vi "Subscriber.vi"() -> ()   [LabVIEW 2020]
panel:
  in  "stop":bool
  out "String":string
  out "Numeric":dbl
  out "Boolean":bool
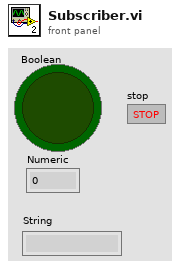
[diagram p1: front panel]
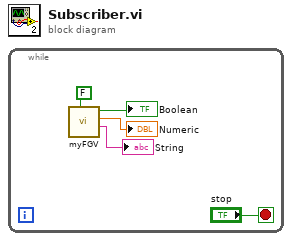
[diagram p0: block diagram]
diagram:
  n1 = while {
    stop <- "stop" stop-if-true
    n2 = call "myFGV.vi"("P/S?"=FALSE) -> ("String"=→"String":string, "Numeric"=→"Numeric":dbl, "Boolean"=→"Boolean":bool)  [unwired: 8 in]
  }
